vi "CANOpen_Search Channel Refs.vi"(8 "error in (no error)":errorcluster, 9 "GUID":string, 10 "Section Ref in":T2 format="%.0x", 11 "Device Ref":T2 format="%.0x") -> (0 "error out":errorcluster, 2 "Found":bool, 3 "Channel Data References":T1[](array[typedef]) format="%.0x")   [LabVIEW 2013, in "CANOpen Addon Custom Device.lvlib"]
uses:
  CANOpen Addon Custom Device.lvlib
  <vilib>/NI Veristand/Custom Device API/Custom Device Item Ref.ctl
  <vilib>/NI Veristand/Custom Device API/Data Reference.ctl
  <vilib>/NI Veristand/Custom Device API/Data Access Type.ctl
  <vilib>/NI Veristand/Custom Device Tools/Custom Device Utility Library/NI VeriStand - Search for All Items by GUID.vi
  <vilib>/NI VeriStand/Custom Device Tools/Custom Device Utility Library/Custom Device Utility Library.lvlib
  <vilib>/NI VeriStand/Custom Device API/Custom Device API.lvlib
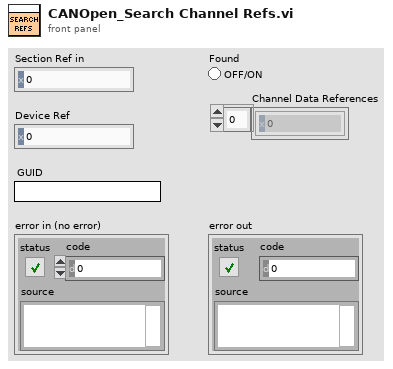
[diagram p1: front panel]
types:
  T1 = typedef "Custom Device API.lvlib/Data Reference.ctl" = i32
  T2 = typedef "Custom Device API.lvlib/Custom Device Item Ref.ctl" = u64
  T3 = typedef "Custom Device API.lvlib/Data Access Type.ctl" = enum16{"Read", "Write"}
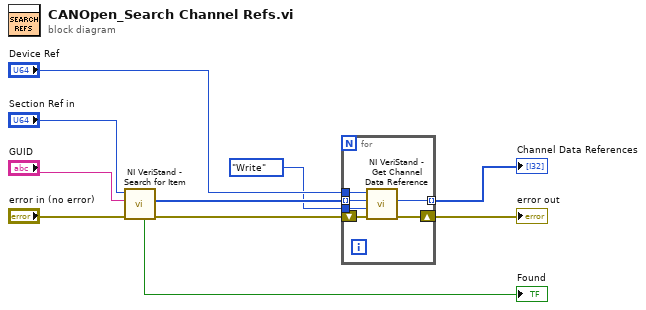
[diagram p0: block diagram]
diagram:
  n1 = call-poly <vilib>:"NI VeriStand - Search for Item.vi"("error in"="error in (no error)", "Item GUID"="GUID", "Section Ref in"="Section Ref in") -> ("error out"=w7:errorcluster, "Item Refs"=w6:T2[], "Found"=→"Found":bool)  [unwired: 5 in, 1 out]
  n2 = for {
    shift-right: [w15] -> w5
    shift-left: w7 -> [w16]
    tunnel: w6 -> [w13] mode=indexing
    tunnel: [w14] -> w3 mode=indexing
    tunnel: "Device Ref" -> [w12]
    tunnel: Data_Access_Type."Write" ("Access") -> [w11]
    n3 = call <vilib>:"NI VeriStand - Get Channel Data Reference.vi"("error in (no error)"=w16, "Access"=w11, "Channel Ref in"=w13, "Device Ref in"=w12) -> ("error out"=w15:errorcluster, "Channel Data Reference"=w14:T1)  [unwired: 5 in, 1 out]
  }
  "error out" <- w5
  "Channel Data References" <- w3
